vi "ContainerNumToBarcode.vi"(8 "error in":errorcluster, 11 "Container num.":i32=2) -> (0 "error out":errorcluster, 1 "Container num. Out":i32=2, 2 "cnt. Barcodes":i32, 3 "Container barcode":string, 4 "Barcode array":string[](array[string]))   [LabVIEW 2024]
panel:
  out "array":string[][](array[string])
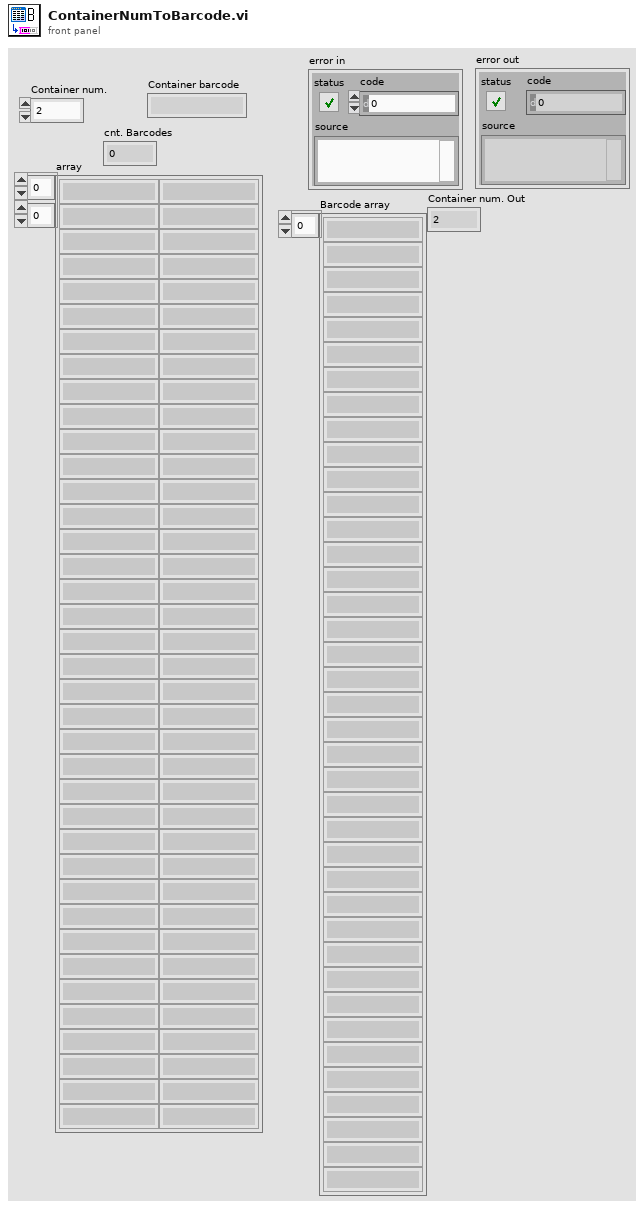
[diagram p1: front panel]
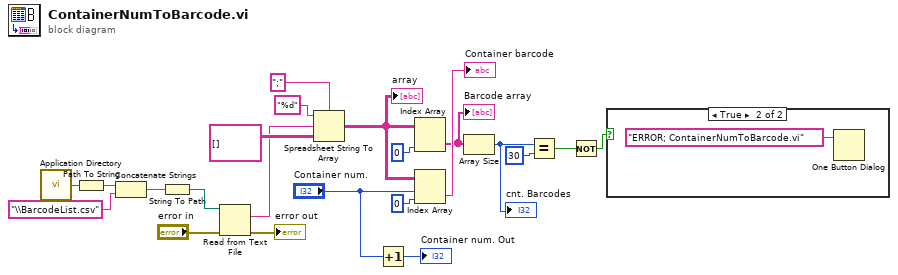
[diagram p0: block diagram]
diagram:
  n1 = call <vilib>:"Application Directory.vi"() -> ("Application Directory"=w10:path)
  n2 = Path To String(path=w10) -> (string=w9:string)
  n3 = Concatenate Strings(w9, "\\BarcodeList.csv" ("string")) -> (w8:string)
  n4 = String To Path(string=w8) -> (path=w6:path)
  n5 = Read from Text File(file (use dialog)=w6, error in="error in") -> (text=w19:string, error out=→"error out":errorcluster)  [unwired: 2 in, 2 out]
  n6 = Spreadsheet String To Array(delimiter (Tab)=";", format string="%d", spreadsheet string=w19, array type (2D Dbl)=string[][] []) -> (array=w16:string[][])
  "array" <- w16
  n7 = Increment(x="Container num.") -> (x+1=→"Container num. Out":i32)
  n8 = Index Array(array=w16, index (col)=0 ("disabled index (col)")) -> (element=w14:string[])  [unwired: 1 in]
  "Barcode array" <- w14
  n9 = Index Array(array=w16, index (row)="Container num.", index (col)=0 ("disabled index (col)")) -> (element=→"Container barcode":string)
  n10 = Array Size(array=w14) -> (size(s)=w12:i32)
  "cnt. Barcodes" <- w12
  n11 = Equal?(x=w12, y=30) -> (x = y?=w11:bool)
  n12 = Not(x=w11) -> (.not. x?=w3:bool)
  n13 = case shown="True" w3 {
    frame False {
    }
    frame True {
      n14 = One Button Dialog(message="ERROR; ContainerNumToBarcode.vi" ("string")) -> ()  [unwired: 1 in, 1 out]
    }
  }
